vi "Client Type.vi"(8 "error in (no error)":errorcluster, 11 "TcpResource in":refnum<class "TcpResource.lvclass">) -> (0 "error out":errorcluster, 2 "Client":refnum<class "Connection.lvclass">, 3 "TcpResource out":refnum<class "TcpResource.lvclass">)   [LabVIEW 2020, in "PicoG-Core.lvlib" / "TcpResource.lvclass"]
uses:
  TcpResource.lvclass
  TcpResource.lvclass/TcpResource.ctl
  <vilib>/IlluminatedG/lv-stream-tcp/TCP Client/TCP Client.lvclass
  C:/Program Files (x86)/National Instruments/LabVIEW 2020/vi.lib/IlluminatedG/lv-stream/Connection/Connection.lvclass
  C:/Program Files (x86)/National Instruments/LabVIEW 2020/vi.lib/IlluminatedG/lv-stream/Endpoint/Endpoint.lvclass
  C:/Program Files (x86)/National Instruments/LabVIEW 2020/vi.lib/IlluminatedG/lv-stream-tcp/TCP Client/TCP Client.lvclass
  <vilib>/IlluminatedG/lv-stream/Connection/Connection.lvclass
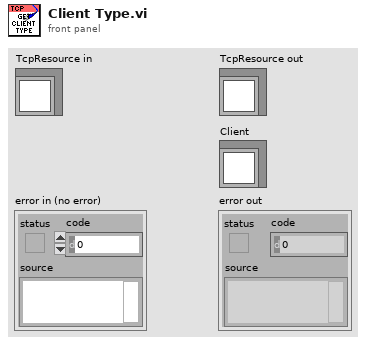
[diagram p1: front panel]
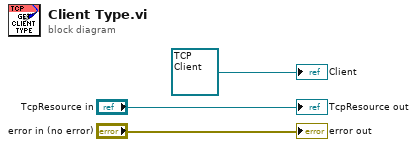
[diagram p0: block diagram]
diagram:
  "error out" <- "error in (no error)"
  "TcpResource out" <- "TcpResource in"
  "Client" <- refnum<class "TCP Client.lvclass"> refnum ("TCP Client in")
